vi "CLSUIP_SaveArrayIndexOfReplacement.vi"(3 "Terminal Index":u32, 4 "Terminal.IsSource":bool, 5 "ElementWrapperRetooler in":refnum<class "ElementWrapperRetooler.lvclass">) -> (2 "ElementWrapperRetooler out":refnum<class "ElementWrapperRetooler.lvclass">)   [LabVIEW 2021, in "MemberVICreation.lvlib" / "ElementWrapperRetooler.lvclass"]
uses:
  <resource>/Framework/Providers/LVClassLibrary/NewAccessors/ElementWrapperRetooler/ElementWrapperRetooler.lvclass
  <resource>/Framework/Providers/LVClassLibrary/NewAccessors/ElementWrapperRetooler/ElementWrapperRetooler.lvclass/ElementWrapperRetooler.ctl
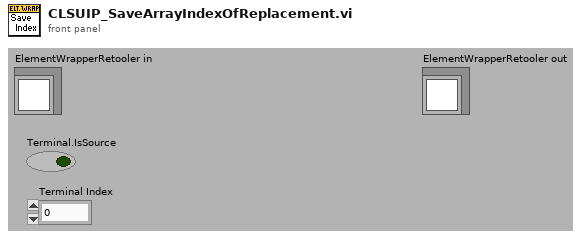
[diagram p1: front panel]
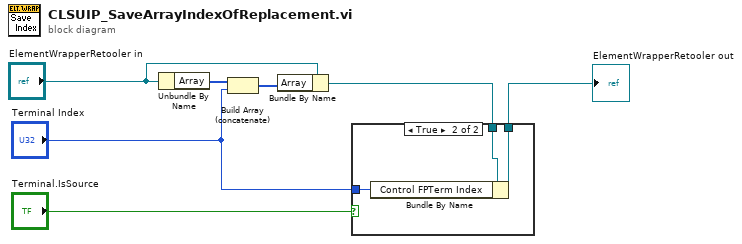
[diagram p0: block diagram]
diagram:
  n1 = Unbundle By Name("ElementWrapperRetooler in") -> ("Array"=w6:u32[])
  n2 = Build Array (concatenate)(w6, "Terminal Index") -> (w5:u32[])
  n3 = Bundle By Name(cluster="ElementWrapperRetooler in", "Array"=w5) -> (w3:refnum<class "ElementWrapperRetooler.lvclass">)
  n4 = case shown="True" "Terminal.IsSource" {
    tunnel: w3 -> [w8 w11]
    tunnel: [w8 w10] -> w2
    tunnel: "Terminal Index" -> [_ w9]
    frame False {
    }
    frame True {
      n5 = Bundle By Name(cluster=w11, "Control FPTerm Index"=w9) -> (w10:refnum<class "ElementWrapperRetooler.lvclass">)
    }
  }
  "ElementWrapperRetooler out" <- w2
